vi "Event Notification.Decide when to Notify.vi"(4 "IsNotControlRef":bool, 6 "IsEmptyStr":bool, 7 "Sys Level":T1, 8 "error in":errorcluster, 9 "Display":bool, 10 "Log":bool, 11 "Level":T1 caption="Notification Level") -> (1 "Display":bool, 2 "Log":bool, 3 "Fwd to Parent":bool)   [LabVIEW 2024, in "EQMF.lvlib" / "Event Log.lvlib"]
uses:
  Event Log.lvlib
  Event Log.Log Level.ctl
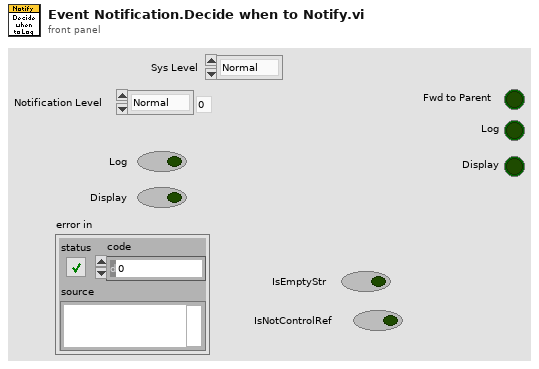
[diagram p1: front panel]
types:
  T1 = typedef "EQMF.lvlib/Event Log.lvlib/Event Log.Log Level.ctl" = enum16{"Normal", "Verbose", "Debug0", "Debug1", "Debug2"}
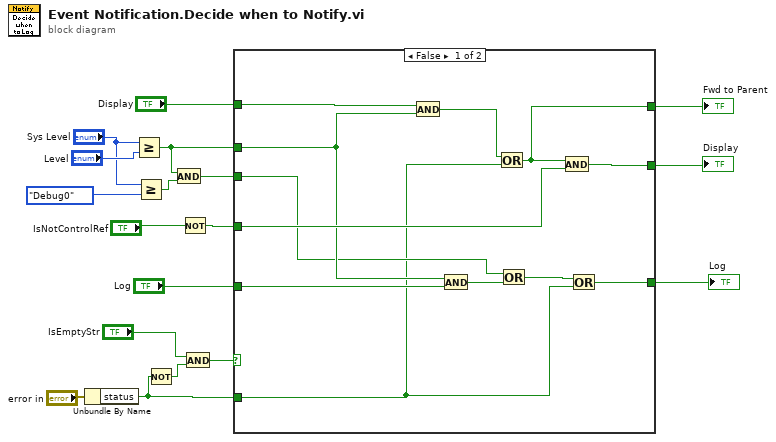
[diagram p0: block diagram]
diagram:
  n1 = Unbundle By Name("error in") -> ("status"=w6:bool)
  n2 = Greater Or Equal?(x="Sys Level", y="Level") -> (x >= y?=w14:bool)
  n3 = Greater Or Equal?(x="Sys Level", y=Event_Log.Log_Level."Debug0" ("Level")) -> (x >= y?=w15:bool)
  n4 = Not(x=w6) -> (.not. x?=w7:bool)
  n5 = And(x=w14, y=w15) -> (x .and. y?=w13:bool)
  n6 = Not(x="IsNotControlRef") -> (.not. x?=w3:bool)
  n7 = And(x="IsEmptyStr", y=w7) -> (x .and. y?=w1:bool)
  n8 = case shown="False" w1 {
    tunnel: w3 -> [w30 _]
    tunnel: [w28 _] -> w18
    tunnel: "Display" -> [w29 _]
    tunnel: w14 -> [w27 _]
    tunnel: w13 -> [w24 _]
    tunnel: [w19 _] -> w12
    tunnel: "Log" -> [w26 _]
    tunnel: [w22 _] -> w10
    tunnel: w6 -> [w20 _]
    frame False {
      n9 = And(x=w29, y=w27) -> (x .and. y?=w21:bool)
      n10 = And(x=w27, y=w26) -> (x .and. y?=w25:bool)
      n11 = Or(x=w21, y=w20) -> (x .or. y?=w19:bool)
      n12 = Or(x=w24, y=w25) -> (x .or. y?=w23:bool)
      n13 = And(x=w19, y=w30) -> (x .and. y?=w28:bool)
      n14 = Or(x=w23, y=w20) -> (x .or. y?=w22:bool)
    }
    frame True {
      # "Nothing to Log"
    }
  }
  "Fwd to Parent" <- w12
  "Display" <- w18
  "Log" <- w10
